vi "To Waveform.vi"(8 "error in (no error)":errorcluster, 11 "Time Stamp Array in":refnum<class "Time Stamp Array.lvclass">) -> (0 "error out":errorcluster, 1 "Success?":bool, 3 "Waveform Array":waveform(dbl)[](array[waveform]))   [LabVIEW 2020, in "Data.lvlib" / "Time Stamp Array.lvclass"]
doc: "Interpret 'Data' as a Waveform Array. If impossible 'Success?' is set to FALSE"
uses:
  Time Stamp Array.lvclass
  Time Stamp Array.lvclass/Time Stamp Array.ctl
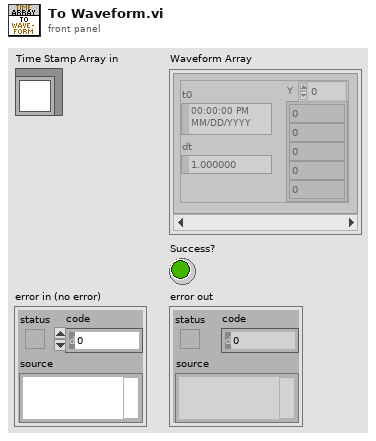
[diagram p1: front panel]
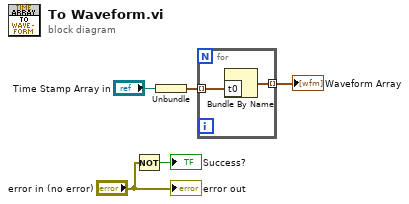
[diagram p0: block diagram]
diagram:
  n1 = Not(x="error in (no error)") -> (.not. x?=→"Success?":bool)
  n2 = Unbundle("Time Stamp Array in") -> (w4:timestamp[])
  n3 = for {
    tunnel: w4 -> [w7] mode=indexing
    tunnel: [w6] -> w1 mode=indexing
    n4 = Bundle By Name("t0"=w7) -> (w6:waveform(dbl))  [unwired: 1 in]
  }
  "Waveform Array" <- w1
  "error out" <- "error in (no error)"
